vi "AT Get Int Max A.vi"(8 "error in (no error)":errorcluster, 10 "Feature":string, 11 "Handle":i32) -> (0 "error out":errorcluster, 2 "MaxValue":i64, 3 "Status":i32)   [LabVIEW 2009]
doc: "Get Int Max\n\nOutput:\n I32 Status\n I64 Max value\n\nInput:\n I32 Handle\n String Feature\n\nThis function will return the maximum allowable value for the specified integer type feature."
uses:
  atcoreA.dll
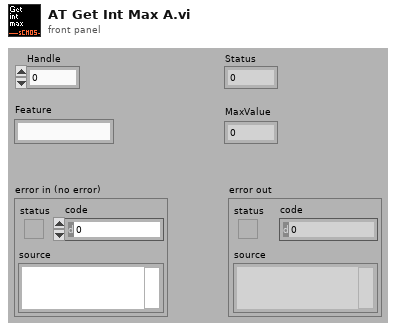
[diagram p1: front panel]
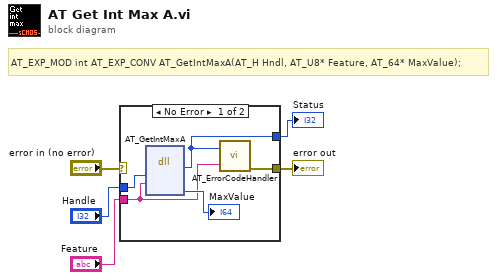
[diagram p0: block diagram]
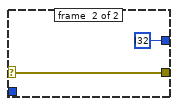
[diagram p2: hidden frame]
diagram:
  # "AT_EXP_MOD int AT_EXP_CONV AT_GetIntMaxA(AT_H Hndl, AT_U8* Feature, AT_64* MaxValue);"
  n1 = case shown="No Error" "error in (no error)" {
    selector: "error in (no error)" -> [_ w12]
    tunnel: [w7 i32 ?] -> w5
    tunnel: "Handle" -> [w10 _]
    tunnel: "Feature" -> [w6 _]
    tunnel: [w8 w12] -> w1
    frame #0 {
      n2 = dll-call lib="atcoreA.dll" fn="AT_GetIntMaxA"("Handle"=w10, "Feature"=w6) -> ("Status"=w7:i32, "MaxValue"=→"MaxValue":i64)  [unwired: 6 in, 2 out]
      n3 = call "AT_ErrorCodeHandler.vi"("Error"=w7, "Feature Name"=w6) -> ("error out"=w8:errorcluster)  [unwired: 5 in]
    }
    frame #1 {
    }
  }
  "Status" <- w5
  "error out" <- w1
